vi "clamp2.vi"(0 "Image In":T1, 7 "error in":errorcluster) -> (20 "Image Out":T1, 27 "error out":errorcluster)   [LabVIEW 2013]
uses:
  <vilib>/vision/Image Controls.llb/IMAQ Image.ctl
  <vilib>/vision/Measure.llb/Edge Options.ctl
  <vilib>/vision/Measure.llb/Edge Polarity.ctl
  <vilib>/vision/NI_Vision_Development_Module.lvlib
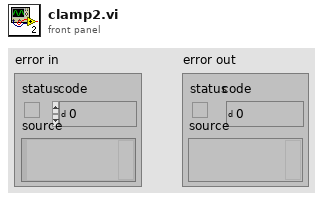
[diagram p1: front panel]
types:
  T1 = typedef "IMAQ Image.ctl" = refnum<image>
  T2 = cluster{"Contrast":i32, "Filter width":i32, "Steepness":i32, "Subsampling Ratio":u32, "Show Search Area":bool, "Show Search Lines":bool, "Show Edges Found":bool, "Show Result":bool}
  T3 = cluster{"Global Rectangle":i32[], "Contours":cluster{"ID":enum32{"External", "Internal"}, "Type":u32, "Coordinates":i32[]}[]}
  T4 = typedef "Edge Options.ctl" = cluster{"Edge Polarity":T5, "Kernel Size":u32, "Width":u32, "Minimum Edge Strength":sgl, "Interpolation Type":enum32{"Zero Order", "Bilinear", "Quadratic", "Cubic", "Bilinear Fixed"}, "Data Processing Method":enum32{"Average", "Median"}}
  T5 = typedef "Edge Polarity.ctl" = u32
  T6 = cluster{"Search  Direction":u32, "Edge Options":T4, "Show Search Area":bool, "Show Search Lines":bool, "Show Edges Found":bool, "Show Result":bool, "Search Area Color":u32, "Search Lines Color":u32, "Edge Locations Color":u32, "Result Color":u32, "Overlay Group Name":string}
  T7 = cluster{"Process":enum16{"Get First Edge", "Get First + Last Edge", "Get All Edges", "Get Best Edge"}, "Step Size":i32, "Max Pixel Radius":i32}
  T8 = cluster{"Center (Pixels)":cluster{"X":sgl, "Y":sgl}, "Radius (Pixels)":dbl, "Center (Real-World)":cluster{"X":sgl, "Y":sgl}, "Radius (Real-World)":dbl, "Roundness (Real-World)":dbl, "Average Strength":dbl, "Average SNR (dB)":dbl}
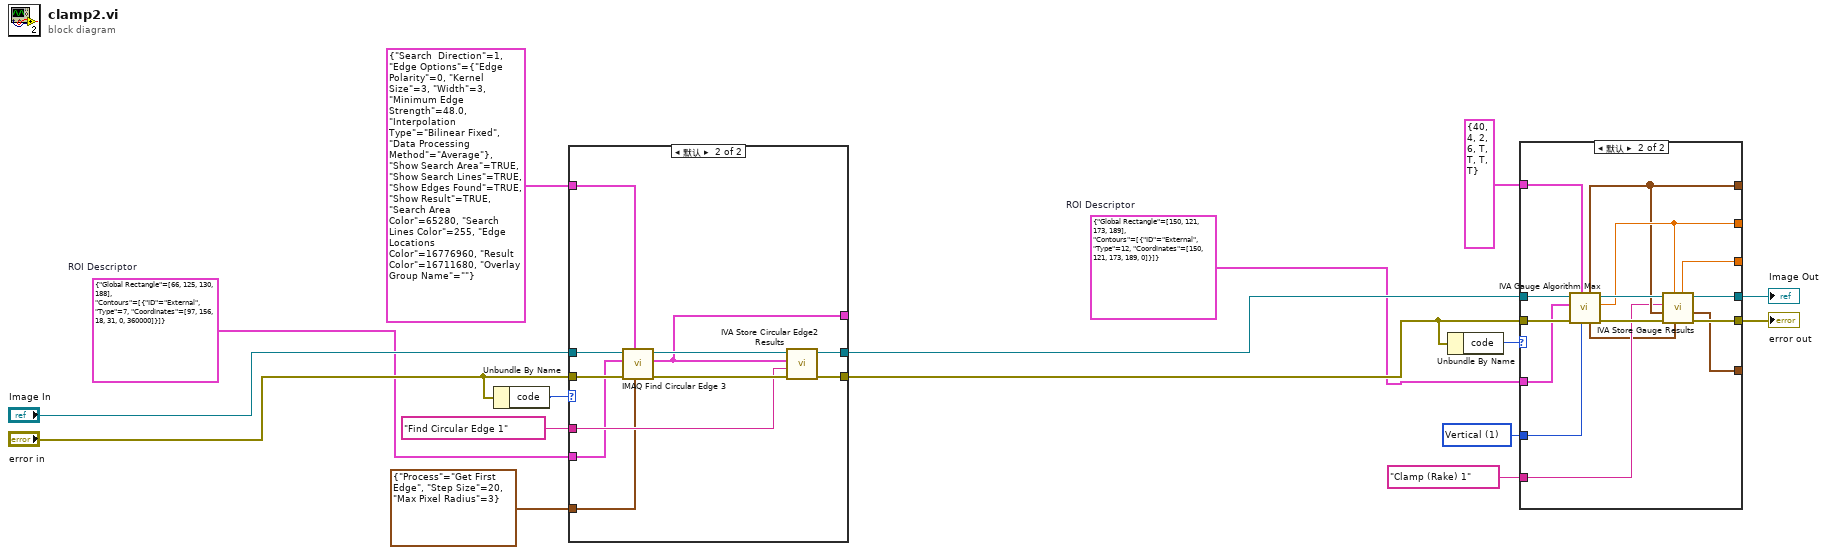
[diagram p0: block diagram]
diagram:
  w6 = u32 1 items=["Horizontal", "Vertical"] ("Scanning axis")
  w5 = T3 {"Global Rectangle"=[150, 121, 173, 189], "Contours"=[{"ID"=enum."External", "Type"=12, "Coordinates"=[150, 121, 173, 189, 0]}]}  # ROI Descriptor
  w12 = T3 {"Global Rectangle"=[66, 125, 130, 188], "Contours"=[{"ID"=enum."External", "Type"=7, "Coordinates"=[97, 156, 18, 31, 0, 360000]}]}  # ROI Descriptor
  n1 = Unbundle By Name("error in") -> ("code"=w11:i32)
  n2 = case "条件结构" shown="默认" w11 {
    tunnel: T6 {"Search  Direction"=1, "Edge Options"={"Edge Polarity"=0, "Kernel Size"=3, "Width"=3, "Minimum Edge Strength"=48.0, "Interpolation Type"=enum."Bilinear Fixed", "Data Processing Method"=enum."Average"}, "Show Search Area"=TRUE, "Show Search Lines"=TRUE, "Show Edges Found"=TRUE, "Show Result"=TRUE, "Search Area Color"=65280, "Search Lines Color"=255, "Edge Locations Color"=16776960, "Result Color"=16711680, "Overlay Group Name"=""} ("Options") -> [_ w18]
    tunnel: "Image In" -> [w17 w28]
    tunnel: "error in" -> [_ w27]
    tunnel: [_ w25] -> w14
    tunnel: [w17 w23] -> w8
    tunnel: "Find Circular Edge 1" ("Step Name") -> [_ w22]
    tunnel: w12 -> [_ w21]
    tunnel: T7 {"Process"=enum."Get First Edge", "Step Size"=20, "Max Pixel Radius"=3} ("Circle Fit Options") -> [_ w20]
    tunnel: [_ w19] -> _
    frame -1074396199, -1074396198 {
      # "Discard Coordinate System Error"
    }
    frame Default {
      n3 = call "IMAQ Find Circular Edge 3"("Circle Fit Options"=w20, "Options"=w18, "error in (no error)"=w27, "ROI Descriptor"=w21, "Image"=w28) -> ("error out"=w26:errorcluster, "Fitted Circle"=w19:T8, "Image Out"=w24:T1)  [unwired: 2 in, 2 out]
      n4 = call <vilib>:"IVA Store Circular Edge2 Results.vi"("error in (no error)"=w26, "Step Name"=w22, "Fitted Circle"=w19, "Image in"=w24) -> ("error out"=w25:errorcluster, "Image dup"=w23:T1)  [unwired: 2 in, 4 out]
    }
  }
  n5 = Unbundle By Name(w14) -> ("code"=w2:i32)
  n6 = case "条件结构" shown="默认" w2 {
    tunnel: w8 -> [w29 w44]
    tunnel: w14 -> [_ w43]
    tunnel: T2 {"Contrast"=40, "Filter width"=4, "Steepness"=2, "Subsampling Ratio"=6, "Show Search Area"=TRUE, "Show Search Lines"=TRUE, "Show Edges Found"=TRUE, "Show Result"=TRUE} ("Settings") -> [_ w42]
    tunnel: w6 -> [_ w41]
    tunnel: w5 -> [_ w40]
    tunnel: [w29 w38] -> w4
    tunnel: [_ w36] -> w3
    tunnel: [_ w35] -> _
    tunnel: [_ w34] -> _
    tunnel: [_ w33] -> _
    tunnel: [_ w32] -> _
    tunnel: "Clamp (Rake) 1" ("Step Name") -> [_ w31]
    frame -1074396199, -1074396198 {
      # "Discard Coordinate System Error"
    }
    frame Default {
      n7 = call <vilib>:"IVA Gauge Algorithm Max.vi"("Scanning axis"=w41, "Settings"=w42, "error in (no error)"=w43, "ROI Descriptor"=w40, "Image"=w44) -> ("error out"=w37:errorcluster, "Distance"=w35:sgl, "Image Out"=w39:T1, "Distance Points"=w30:cluster{"X":sgl, "Y":sgl}[], "Points of Contact"=w34:cluster{"X":sgl, "Y":sgl}[])  [unwired: 1 in, 1 out]
      n8 = call <vilib>:"IVA Store Gauge Results.vi"("Distance Points"=w30, "Distance"=w35, "error in (no error)"=w37, "Points of Contact"=w34, "Step Name"=w31, "Image in"=w39) -> ("error out"=w36:errorcluster, "Points of Contact (calibrated)"=w32:cluster{"X":sgl, "Y":sgl}[], "Image dup"=w38:T1, "Distance (calibrated)"=w33:sgl)  [unwired: 2 out]
    }
  }
  "Image Out" <- w4
  "error out" <- w3
